vi "set default value.vi"(11 "tag":refnum<class "tag descriptor.lvclass">) -> (1 "cancelled?":bool, 3 "tag out":refnum<class "tag descriptor.lvclass">)   [LabVIEW 2013, in "fixed channel tag bus module editor node.lvclass"]
uses:
  fixed channel tag bus module editor node.lvclass
  <vilib>/NI/Tag Bus/tag/tag descriptor.lvclass
  <vilib>/NI/Tag Bus/tag/Data Type.ctl
  <vilib>/NI/Tag Bus/tag/tag descriptor.lvclass/tag descriptor.ctl
  <vilib>/NI/Tag Bus/tag/read tag name.vi
  <vilib>/NI/Tag Bus/tag/default value polymorphs/read default value Double.vi
  <vilib>/NI/Tag Bus/tag/default value polymorphs/read default value Single.vi
  <vilib>/NI/Tag Bus/tag/default value polymorphs/read default value I64.vi
  <vilib>/NI/Tag Bus/tag/default value polymorphs/read default value I32.vi
  <vilib>/NI/Tag Bus/tag/default value polymorphs/read default value I16.vi
  <vilib>/NI/Tag Bus/tag/default value polymorphs/read default value I8.vi
  <vilib>/NI/Tag Bus/tag/default value polymorphs/read default value U64.vi
  <vilib>/NI/Tag Bus/tag/default value polymorphs/read default value U32.vi
  <vilib>/NI/Tag Bus/tag/default value polymorphs/read default value U16.vi
  <vilib>/NI/Tag Bus/tag/default value polymorphs/read default value U8.vi
  <vilib>/NI/Tag Bus/tag/default value polymorphs/read default value String.vi
  <vilib>/NI/Tag Bus/tag/default value polymorphs/read default value Boolean.vi
  <vilib>/NI/Tag Bus/tag/default value polymorphs/read default value Array of U8.vi
  <vilib>/NI/Tag Bus/tag/default value polymorphs/read default value Array of U16.vi
  <vilib>/NI/Tag Bus/tag/default value polymorphs/read default value Array of U32.vi
  <vilib>/NI/Tag Bus/tag/default value polymorphs/read default value Array of U64.vi
  <vilib>/NI/Tag Bus/tag/default value polymorphs/read default value Array of I64.vi
  <vilib>/NI/Tag Bus/tag/default value polymorphs/read default value Array of I32.vi
  <vilib>/NI/Tag Bus/tag/default value polymorphs/read default value Array of I16.vi
  <vilib>/NI/Tag Bus/tag/default value polymorphs/read default value Array of I8.vi
  <vilib>/NI/Tag Bus/tag/default value polymorphs/read default value Array of Double.vi
  <vilib>/NI/Tag Bus/tag/default value polymorphs/read default value Array of Single.vi
  <vilib>/NI/Tag Bus/tag/default value polymorphs/read default value Array of Boolean.vi
  <vilib>/NI/Tag Bus/tag/default value polymorphs/read default value Array of String.vi
  <vilib>/NI/Tag Bus/tag/default value polymorphs/write default value Double.vi
  <vilib>/NI/Tag Bus/tag/default value polymorphs/write default value Single.vi
  <vilib>/NI/Tag Bus/tag/default value polymorphs/write default value String.vi
  <vilib>/NI/Tag Bus/tag/default value polymorphs/write default value Boolean.vi
  <vilib>/NI/Tag Bus/tag/default value polymorphs/write default value Array of U8.vi
  <vilib>/NI/Tag Bus/tag/default value polymorphs/write default value Array of U16.vi
  <vilib>/NI/Tag Bus/tag/default value polymorphs/write default value Array of U32.vi
  <vilib>/NI/Tag Bus/tag/default value polymorphs/write default value Array of U64.vi
  <vilib>/NI/Tag Bus/tag/default value polymorphs/write default value Array of I64.vi
  <vilib>/NI/Tag Bus/tag/default value polymorphs/write default value Array of I32.vi
  <vilib>/NI/Tag Bus/tag/default value polymorphs/write default value Array of I16.vi
  <vilib>/NI/Tag Bus/tag/default value polymorphs/write default value Array of I8.vi
  <vilib>/NI/Tag Bus/tag/default value polymorphs/write default value Array of Double.vi
  <vilib>/NI/Tag Bus/tag/default value polymorphs/write default value Array of Single.vi
  <vilib>/NI/Tag Bus/tag/default value polymorphs/write default value Array of String.vi
  <vilib>/NI/Tag Bus/tag/default value polymorphs/write default value Array of Boolean.vi
  <vilib>/NI/Tag Bus/tag/default value polymorphs/write default value I64.vi
  <vilib>/NI/Tag Bus/tag/default value polymorphs/write default value I32.vi
  <vilib>/NI/Tag Bus/tag/default value polymorphs/write default value I16.vi
  <vilib>/NI/Tag Bus/tag/default value polymorphs/write default value I8.vi
  <vilib>/NI/Tag Bus/tag/default value polymorphs/write default value U64.vi
  <vilib>/NI/Tag Bus/tag/default value polymorphs/write default value U32.vi
  <vilib>/NI/Tag Bus/tag/default value polymorphs/write default value U16.vi
  <vilib>/NI/Tag Bus/tag/default value polymorphs/write default value U8.vi
panel:
  out "data type":T1
  in  "numeric type":ext caption="Default Double"
  in  "string type":string
  in  "boolean type":bool
  in  "numeric array type":ext[](array[numeric])
  in  "string array type":string[](array[string])
  in  "boolean array type":bool[](array[boolean])
  out "Tag Name":string
  in  "Cancel Button":bool
  in  "Save Button":bool
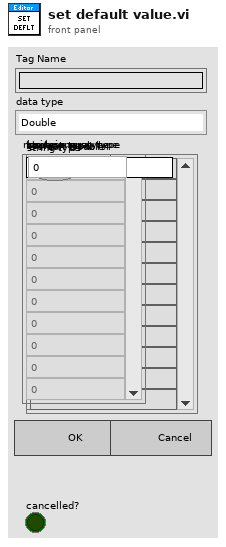
[diagram p1: front panel]
types:
  T1 = typedef "tag bus.lvlib/tag descriptor.lvclass/Data Type.ctl" = enum16{"Double", "Single", "I64", "I32", "I16", "I8", "U64", "U32", "U16", "U8", "Boolean", "String", "Array of Double", "Array of Single", "Array of I64", "Array of I32", "Array of I16", "Array of I8", "Array of U64", "Array of U32", "Array of U16", "Array of U8", "Array of Boolean", "Array of String"}
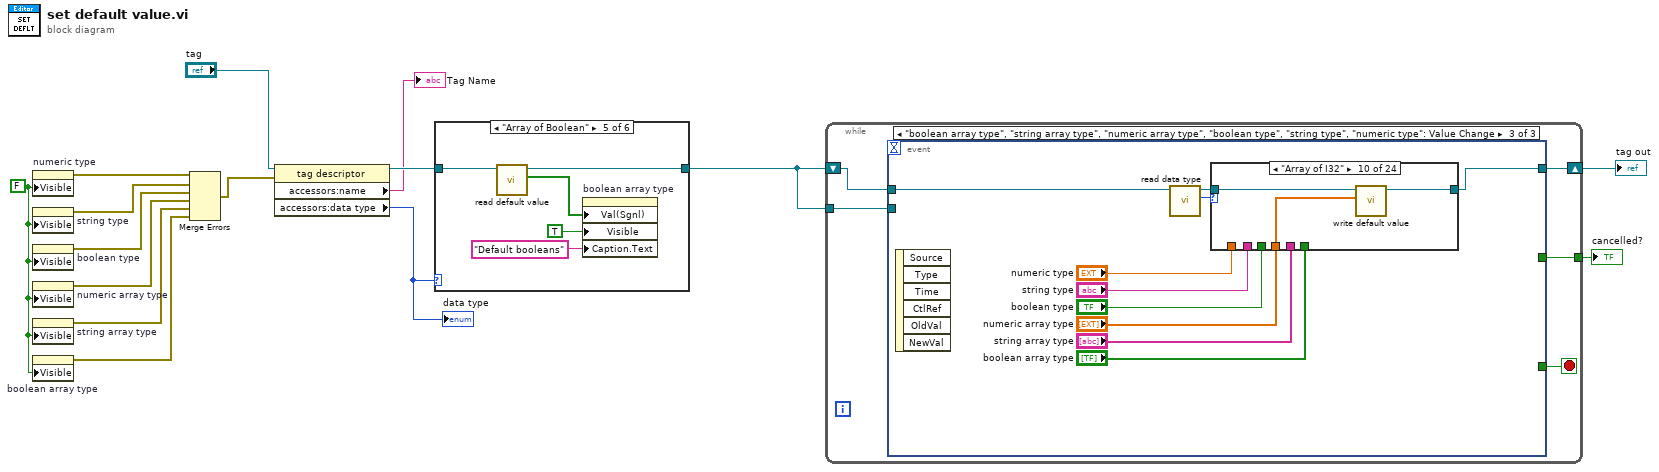
[diagram p0: block diagram]
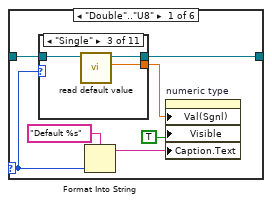
[diagram p2: hidden frame]
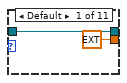
[diagram p3: hidden frame]
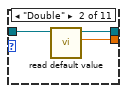
[diagram p4: hidden frame]
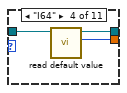
[diagram p5: hidden frame]
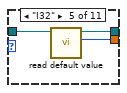
[diagram p6: hidden frame]
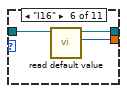
[diagram p7: hidden frame]
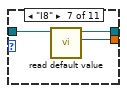
[diagram p8: hidden frame]
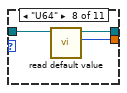
[diagram p9: hidden frame]
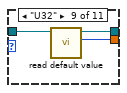
[diagram p10: hidden frame]
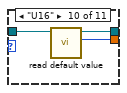
[diagram p11: hidden frame]
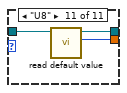
[diagram p12: hidden frame]
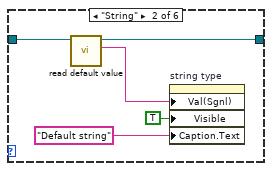
[diagram p13: hidden frame]
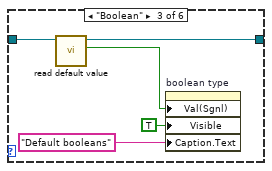
[diagram p14: hidden frame]
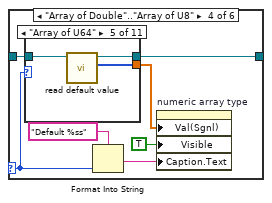
[diagram p15: hidden frame]
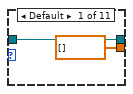
[diagram p16: hidden frame]
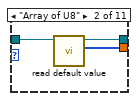
[diagram p17: hidden frame]
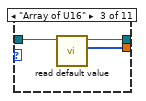
[diagram p18: hidden frame]
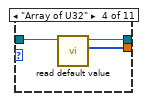
[diagram p19: hidden frame]
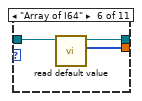
[diagram p20: hidden frame]
diagram:
  w10 = FALSE ("Visible")
  (unwired) TRUE ("Value (Signaling)")
  n1 = property on="numeric type" class="DigNum (strict)"("Visible"=w10) -> (error out=w9:errorcluster)  [unwired: 2 in, 1 out]
  n2 = property on="string type" class="Str"("Visible"=w10) -> (error out=w8:errorcluster)  [unwired: 2 in, 1 out]
  n3 = property on="boolean type" class="Bool (strict)"("Visible"=w10) -> (error out=w7:errorcluster)  [unwired: 2 in, 1 out]
  n4 = property on="numeric array type" class="Arr (strict)"("Visible"=w10) -> (error out=w6:errorcluster)  [unwired: 2 in, 1 out]
  n5 = property on="string array type" class="Arr (strict)"("Visible"=w10) -> (error out=w5:errorcluster)  [unwired: 2 in, 1 out]
  n6 = property on="boolean array type" class="Arr (strict)"("Visible"=w10) -> (error out=w4:errorcluster)  [unwired: 2 in, 1 out]
  n7 = Merge Errors(w9, w8, w7, w6, w5, w4) -> (w3:errorcluster)
  n8 = property class="tag descriptor"(reference="tag", error in=w3) -> (reference out=w13:refnum<class "tag descriptor.lvclass">, "accessors:name"=→"Tag Name":string, "accessors:data type"=w12:T1)  [unwired: 1 out]
  "data type" <- w12
  n9 = case shown="\"Array of Boolean\"" w12 {
    selector: w12 -> [w16 _ _ w65 _ _]
    tunnel: w13 -> [w19 w57 w62 w68 w106 w111]
    tunnel: [w18 w56 w61 w67 w105 w109] -> w2
    frame "Double".."U8" {
      n10 = case shown="\"Single\"" w16 {
        tunnel: w19 -> [w24 w27 w30 w33 w36 w39 w42 w45 w48 w51 w54]
        tunnel: [w24 w26 w29 w32 w35 w38 w41 w44 w47 w50 w53] -> w18
        tunnel: [ext 0.0 ("default value") w25 w28 w31 w34 w37 w40 w43 w46 w49 w52] -> w17
        frame Default {
        }
        frame "Double" {
          n11 = call-poly <vilib>:"read default value.vi"("system tag in"=w27) -> ("default value"=w25:dbl, "system tag out"=w26:refnum<class "tag descriptor.lvclass">)  [unwired: 7 in, 2 out]
        }
        frame "Single" {
          n12 = call-poly <vilib>:"read default value.vi"("system tag in"=w30) -> ("default value"=w28:sgl, "system tag out"=w29:refnum<class "tag descriptor.lvclass">)  [unwired: 7 in, 2 out]
        }
        frame "I64" {
          n13 = call-poly <vilib>:"read default value.vi"("system tag in"=w33) -> ("default value"=w31:i64, "system tag out"=w32:refnum<class "tag descriptor.lvclass">)  [unwired: 7 in, 2 out]
        }
        frame "I32" {
          n14 = call-poly <vilib>:"read default value.vi"("system tag in"=w36) -> ("default value"=w34:i32, "system tag out"=w35:refnum<class "tag descriptor.lvclass">)  [unwired: 7 in, 2 out]
        }
        frame "I16" {
          n15 = call-poly <vilib>:"read default value.vi"("system tag in"=w39) -> ("default value"=w37:i16, "system tag out"=w38:refnum<class "tag descriptor.lvclass">)  [unwired: 7 in, 2 out]
        }
        frame "I8" {
          n16 = call-poly <vilib>:"read default value.vi"("system tag in"=w42) -> ("default value"=w40:i8, "system tag out"=w41:refnum<class "tag descriptor.lvclass">)  [unwired: 7 in, 2 out]
        }
        frame "U64" {
          n17 = call-poly <vilib>:"read default value.vi"("system tag in"=w45) -> ("default value"=w43:u64, "system tag out"=w44:refnum<class "tag descriptor.lvclass">)  [unwired: 7 in, 2 out]
        }
        frame "U32" {
          n18 = call-poly <vilib>:"read default value.vi"("system tag in"=w48) -> ("default value"=w46:u32, "system tag out"=w47:refnum<class "tag descriptor.lvclass">)  [unwired: 7 in, 2 out]
        }
        frame "U16" {
          n19 = call-poly <vilib>:"read default value.vi"("system tag in"=w51) -> ("default value"=w49:u16, "system tag out"=w50:refnum<class "tag descriptor.lvclass">)  [unwired: 7 in, 2 out]
        }
        frame "U8" {
          n20 = call-poly <vilib>:"read default value.vi"("system tag in"=w54) -> ("default value"=w52:u8, "system tag out"=w53:refnum<class "tag descriptor.lvclass">)  [unwired: 7 in, 2 out]
        }
      }
      n21 = Format Into String(format string="Default %s", w16) -> (resulting string=w21:string)  [unwired: 2 in, 1 out]
      n22 = property on="numeric type" class="DigNum (strict)"("Val(Sgnl)"=w17, "Visible"=TRUE, "Caption.Text"=w21) -> ()  [unwired: 2 in, 2 out]
    }
    frame "String" {
      n23 = call-poly <vilib>:"read default value.vi"("system tag in"=w57) -> ("default value"=w55:string, "system tag out"=w56:refnum<class "tag descriptor.lvclass">)  [unwired: 7 in, 2 out]
      n24 = property on="string type" class="Str"("Val(Sgnl)"=w55, "Visible"=TRUE, "Caption.Text"="Default string" ("format string")) -> ()  [unwired: 2 in, 2 out]
    }
    frame "Boolean" {
      n25 = call-poly <vilib>:"read default value.vi"("system tag in"=w62) -> ("default value"=w60:bool, "system tag out"=w61:refnum<class "tag descriptor.lvclass">)  [unwired: 7 in, 2 out]
      n26 = property on="boolean type" class="Bool (strict)"("Val(Sgnl)"=w60, "Visible"=TRUE, "Caption.Text"="Default booleans" ("format string")) -> ()  [unwired: 2 in, 2 out]
    }
    frame "Array of Double".."Array of U8" {
      n27 = case shown="\"Array of U64\"" w65 {
        tunnel: w68 -> [w73 w76 w79 w82 w85 w88 w91 w94 w97 w100 w103]
        tunnel: [w73 w75 w78 w81 w84 w87 w90 w93 w96 w99 w102] -> w67
        tunnel: [ext[] [] ("default value") w74 w77 w80 w83 w86 w89 w92 w95 w98 w101] -> w66
        frame Default {
        }
        frame "Array of U8" {
          n28 = call-poly <vilib>:"read default value.vi"("system tag in"=w76) -> ("default value"=w74:u8[], "system tag out"=w75:refnum<class "tag descriptor.lvclass">)  [unwired: 7 in, 2 out]
        }
        frame "Array of U16" {
          n29 = call-poly <vilib>:"read default value.vi"("system tag in"=w79) -> ("default value"=w77:u16[], "system tag out"=w78:refnum<class "tag descriptor.lvclass">)  [unwired: 7 in, 2 out]
        }
        frame "Array of U32" {
          n30 = call-poly <vilib>:"read default value.vi"("system tag in"=w82) -> ("default value"=w80:u32[], "system tag out"=w81:refnum<class "tag descriptor.lvclass">)  [unwired: 7 in, 2 out]
        }
        frame "Array of U64" {
          n31 = call-poly <vilib>:"read default value.vi"("system tag in"=w85) -> ("default value"=w83:u64[], "system tag out"=w84:refnum<class "tag descriptor.lvclass">)  [unwired: 7 in, 2 out]
        }
        frame "Array of I64" {
          n32 = call-poly <vilib>:"read default value.vi"("system tag in"=w88) -> ("default value"=w86:i64[], "system tag out"=w87:refnum<class "tag descriptor.lvclass">)  [unwired: 7 in, 2 out]
        }
        frame "Array of I32" {
          n33 = call-poly <vilib>:"read default value.vi"("system tag in"=w91) -> ("default value"=w89:i32[], "system tag out"=w90:refnum<class "tag descriptor.lvclass">)  [unwired: 7 in, 2 out]
        }
        frame "Array of I16" {
          n34 = call-poly <vilib>:"read default value.vi"("system tag in"=w94) -> ("default value"=w92:i16[], "system tag out"=w93:refnum<class "tag descriptor.lvclass">)  [unwired: 7 in, 2 out]
        }
        frame "Array of I8" {
          n35 = call-poly <vilib>:"read default value.vi"("system tag in"=w97) -> ("default value"=w95:i8[], "system tag out"=w96:refnum<class "tag descriptor.lvclass">)  [unwired: 7 in, 2 out]
        }
        frame "Array of Double" {
          n36 = call-poly <vilib>:"read default value.vi"("system tag in"=w100) -> ("default value"=w98:dbl[], "system tag out"=w99:refnum<class "tag descriptor.lvclass">)  [unwired: 7 in, 2 out]
        }
        frame "Array of Single" {
          n37 = call-poly <vilib>:"read default value.vi"("system tag in"=w103) -> ("default value"=w101:sgl[], "system tag out"=w102:refnum<class "tag descriptor.lvclass">)  [unwired: 7 in, 2 out]
        }
      }
      n38 = Format Into String(format string="Default %ss", w65) -> (resulting string=w70:string)  [unwired: 2 in, 1 out]
      n39 = property on="numeric array type" class="Arr (strict)"("Val(Sgnl)"=w66, "Visible"=TRUE, "Caption.Text"=w70) -> ()  [unwired: 2 in, 2 out]
    }
    frame "Array of Boolean" {
      n40 = call-poly <vilib>:"read default value.vi"("system tag in"=w106) -> ("default value"=w104:bool[], "system tag out"=w105:refnum<class "tag descriptor.lvclass">)  [unwired: 7 in, 2 out]
      n41 = property on="boolean array type" class="Arr (strict)"("Val(Sgnl)"=w104, "Visible"=TRUE, "Caption.Text"="Default booleans") -> ()  [unwired: 2 in, 2 out]
    }
    frame "Array of String" {
      n42 = call-poly <vilib>:"read default value.vi"("system tag in"=w111) -> ("default value"=w110:string[], "system tag out"=w109:refnum<class "tag descriptor.lvclass">)  [unwired: 7 in, 2 out]
      n43 = property on="string array type" class="Arr (strict)"("Val(Sgnl)"=w110, "Visible"=TRUE, "Caption.Text"="Default strings") -> ()  [unwired: 2 in, 2 out]
    }
  }
  n44 = while {
    tunnel: [w118] -> w1
    shift-right: [w116] -> w14
    shift-left: w2 -> [w115]
    tunnel: w2 -> [w114]
    stop <- w117 stop-if-true
    n45 = event shown="[2] \"boolean array type\", \"string array type\", \"numeric array type\", \"boolean type\", \"string type\", \"numeric type\": Value Change" {
      selector: _ -> [_ _ _]
      dyn-events: _ -> [_ _ _]
      timeout: _ -> [_ _ _]
      tunnel: [_ FALSE _] -> w118
      tunnel: ["Save Button" TRUE _] -> w117
      tunnel: [w119 w121 w125] -> w116
      tunnel: w115 -> [w119 _ w124]
      tunnel: w114 -> [_ w121 _]
      event "Save Button": Value Change {
        n46 = event-data() -> ()  [unwired: 1 in, 6 out]
      }
      event Panel Close; "Cancel Button": Value Change {
        n47 = event-data() -> ()  [unwired: 1 in, 3 out]
      }
      event "boolean array type", "string array type", "numeric array type", "boolean type", "string type", "numeric type": Value Change {
        n48 = event-data() -> ()  [unwired: 1 in, 6 out]
        n49 = call <vilib>:"read data type.vi"("system tag in"=w124) -> ("data type"=w126:T1, "system tag out"=w127:refnum<class "tag descriptor.lvclass">)  [unwired: 8 in, 1 out]
        n50 = case shown="\"Array of I32\"" w126 {
          tunnel: [w136 w139 w142 w145 w148 w151 w154 w157 w160 w163 w166 w169 w172 w175 w178 w181 w184 w187 w190 w193 w196 w199 w202 w205] -> w125
          tunnel: w127 -> [w135 w138 w141 w144 w147 w150 w153 w156 w159 w162 w165 w168 w171 w174 w177 w180 w183 w186 w189 w192 w195 w198 w201 w204]
          tunnel: "numeric type" -> [w134 w137 _ _ _ _ _ _ _ _ _ _ _ _ _ _ w182 w185 w188 w191 w194 w197 w200 w203]
          tunnel: "string type" -> [_ _ w140 _ _ _ _ _ _ _ _ _ _ _ _ _ _ _ _ _ _ _ _ _]
          tunnel: "boolean type" -> [_ _ _ w143 _ _ _ _ _ _ _ _ _ _ _ _ _ _ _ _ _ _ _ _]
          tunnel: "numeric array type" -> [_ _ _ _ w146 w149 w152 w155 w158 w161 w164 w167 w170 w173 _ _ _ _ _ _ _ _ _ _]
          tunnel: "string array type" -> [_ _ _ _ _ _ _ _ _ _ _ _ _ _ w176 _ _ _ _ _ _ _ _ _]
          tunnel: "boolean array type" -> [_ _ _ _ _ _ _ _ _ _ _ _ _ _ _ w179 _ _ _ _ _ _ _ _]
          frame "Double" {
            n51 = call-poly <vilib>:"write default value.vi"("default value"=w134, "system tag in"=w135) -> ("system tag out"=w136:refnum<class "tag descriptor.lvclass">)  [unwired: 8 in, 1 out]
          }
          frame "Single" {
            n52 = call-poly <vilib>:"write default value.vi"("default value"=w137, "system tag in"=w138) -> ("system tag out"=w139:refnum<class "tag descriptor.lvclass">)  [unwired: 8 in, 1 out]
          }
          frame "String" {
            n53 = call-poly <vilib>:"write default value.vi"("default value"=w140, "system tag in"=w141) -> ("system tag out"=w142:refnum<class "tag descriptor.lvclass">)  [unwired: 8 in, 1 out]
          }
          frame "Boolean" {
            n54 = call-poly <vilib>:"write default value.vi"("default value"=w143, "system tag in"=w144) -> ("system tag out"=w145:refnum<class "tag descriptor.lvclass">)  [unwired: 8 in, 1 out]
          }
          frame "Array of U8" {
            n55 = call-poly <vilib>:"write default value.vi"("default value"=w146, "system tag in"=w147) -> ("system tag out"=w148:refnum<class "tag descriptor.lvclass">)  [unwired: 8 in, 1 out]
          }
          frame "Array of U16" {
            n56 = call-poly <vilib>:"write default value.vi"("default value"=w149, "system tag in"=w150) -> ("system tag out"=w151:refnum<class "tag descriptor.lvclass">)  [unwired: 8 in, 1 out]
          }
          frame "Array of U32" {
            n57 = call-poly <vilib>:"write default value.vi"("default value"=w152, "system tag in"=w153) -> ("system tag out"=w154:refnum<class "tag descriptor.lvclass">)  [unwired: 8 in, 1 out]
          }
          frame "Array of U64" {
            n58 = call-poly <vilib>:"write default value.vi"("default value"=w155, "system tag in"=w156) -> ("system tag out"=w157:refnum<class "tag descriptor.lvclass">)  [unwired: 8 in, 1 out]
          }
          frame "Array of I64" {
            n59 = call-poly <vilib>:"write default value.vi"("default value"=w158, "system tag in"=w159) -> ("system tag out"=w160:refnum<class "tag descriptor.lvclass">)  [unwired: 8 in, 1 out]
          }
          frame "Array of I32" {
            n60 = call-poly <vilib>:"write default value.vi"("default value"=w161, "system tag in"=w162) -> ("system tag out"=w163:refnum<class "tag descriptor.lvclass">)  [unwired: 8 in, 1 out]
          }
          frame "Array of I16" {
            n61 = call-poly <vilib>:"write default value.vi"("default value"=w164, "system tag in"=w165) -> ("system tag out"=w166:refnum<class "tag descriptor.lvclass">)  [unwired: 8 in, 1 out]
          }
          frame "Array of I8" {
            n62 = call-poly <vilib>:"write default value.vi"("default value"=w167, "system tag in"=w168) -> ("system tag out"=w169:refnum<class "tag descriptor.lvclass">)  [unwired: 8 in, 1 out]
          }
          frame "Array of Double" {
            n63 = call-poly <vilib>:"write default value.vi"("default value"=w170, "system tag in"=w171) -> ("system tag out"=w172:refnum<class "tag descriptor.lvclass">)  [unwired: 8 in, 1 out]
          }
          frame "Array of Single" {
            n64 = call-poly <vilib>:"write default value.vi"("default value"=w173, "system tag in"=w174) -> ("system tag out"=w175:refnum<class "tag descriptor.lvclass">)  [unwired: 8 in, 1 out]
          }
          frame "Array of String" {
            n65 = call-poly <vilib>:"write default value.vi"("default value"=w176, "system tag in"=w177) -> ("system tag out"=w178:refnum<class "tag descriptor.lvclass">)  [unwired: 8 in, 1 out]
          }
          frame "Array of Boolean" {
            n66 = call-poly <vilib>:"write default value.vi"("default value"=w179, "system tag in"=w180) -> ("system tag out"=w181:refnum<class "tag descriptor.lvclass">)  [unwired: 8 in, 1 out]
          }
          frame "I64" {
            n67 = call-poly <vilib>:"write default value.vi"("default value"=w182, "system tag in"=w183) -> ("system tag out"=w184:refnum<class "tag descriptor.lvclass">)  [unwired: 8 in, 1 out]
          }
          frame "I32" {
            n68 = call-poly <vilib>:"write default value.vi"("default value"=w185, "system tag in"=w186) -> ("system tag out"=w187:refnum<class "tag descriptor.lvclass">)  [unwired: 8 in, 1 out]
          }
          frame "I16" {
            n69 = call-poly <vilib>:"write default value.vi"("default value"=w188, "system tag in"=w189) -> ("system tag out"=w190:refnum<class "tag descriptor.lvclass">)  [unwired: 8 in, 1 out]
          }
          frame "I8" {
            n70 = call-poly <vilib>:"write default value.vi"("default value"=w191, "system tag in"=w192) -> ("system tag out"=w193:refnum<class "tag descriptor.lvclass">)  [unwired: 8 in, 1 out]
          }
          frame "U64" {
            n71 = call-poly <vilib>:"write default value.vi"("default value"=w194, "system tag in"=w195) -> ("system tag out"=w196:refnum<class "tag descriptor.lvclass">)  [unwired: 8 in, 1 out]
          }
          frame "U32" {
            n72 = call-poly <vilib>:"write default value.vi"("default value"=w197, "system tag in"=w198) -> ("system tag out"=w199:refnum<class "tag descriptor.lvclass">)  [unwired: 8 in, 1 out]
          }
          frame "U16" {
            n73 = call-poly <vilib>:"write default value.vi"("default value"=w200, "system tag in"=w201) -> ("system tag out"=w202:refnum<class "tag descriptor.lvclass">)  [unwired: 8 in, 1 out]
          }
          frame "U8" {
            n74 = call-poly <vilib>:"write default value.vi"("default value"=w203, "system tag in"=w204) -> ("system tag out"=w205:refnum<class "tag descriptor.lvclass">)  [unwired: 8 in, 1 out]
          }
        }
      }
    }
  }
  "tag out" <- w14
  "cancelled?" <- w1
